vi "GDSLvClass_GetClassProviderInformation.vi"(0 "Class Refnum In":refnum<vi>, 5 "error in (no error)":errorcluster) -> (14 "Class Refnum Out":refnum<vi>, 15 "ClassProvider":T1, 19 "error out":errorcluster)   [LabVIEW 2020]
uses:
  GDSLvClass_ProviderTypes.ctl
  GDSLvClass_ClassTypeSettingNames.ctl
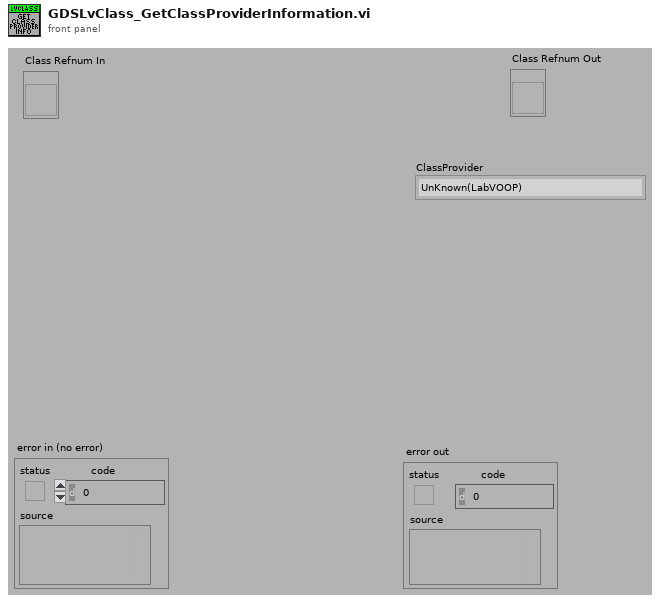
[diagram p1: front panel]
types:
  T1 = typedef "GDSLvClass_ProviderTypes.ctl" = enum16{"UnKnown(LabVOOP)", "Native", "EndevoGOOP3", "OpenG(RootObject)", "OpenG(OpenG_Object)", "EndevoGOOP4", "JKI1"}
  T2 = typedef "GDSLvClass_ClassTypeSettingNames.ctl" = enum16{"EndevoGOOP_ClassProvider", "EndevoGOOP_TemplateUsed", "EndevoGOOP_TemplateVersion", "EndevoGOOP_PlugIns", "EndevoGOOP_ConnectorPanePattern"}
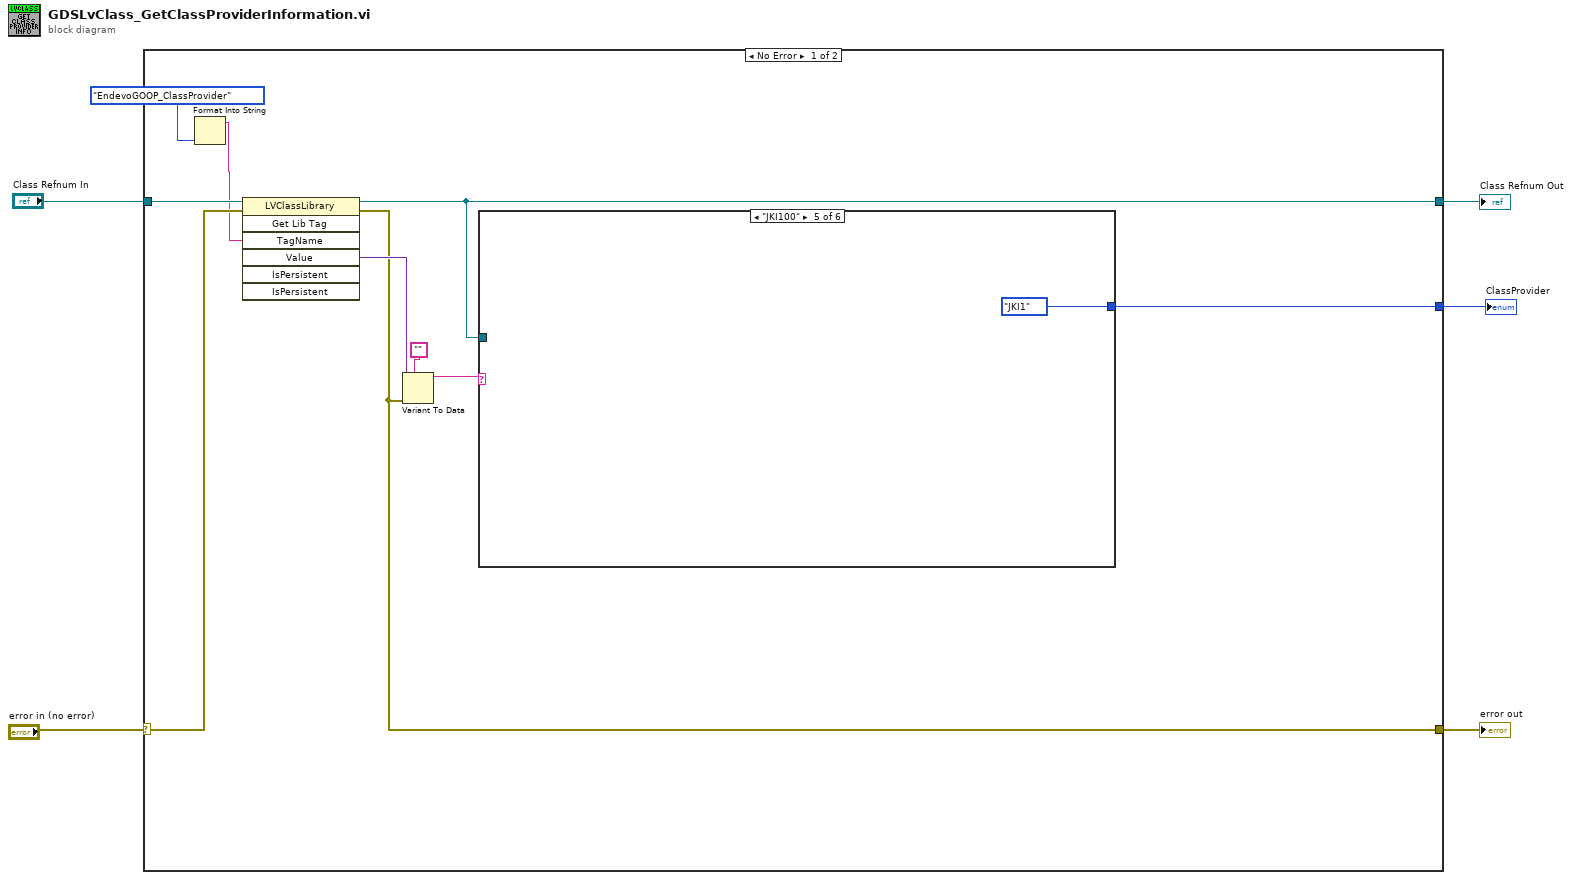
[diagram p0: block diagram]
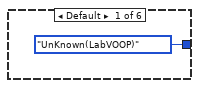
[diagram p2: hidden frame]
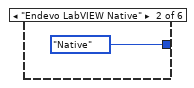
[diagram p3: hidden frame]
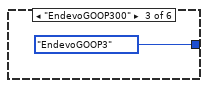
[diagram p4: hidden frame]
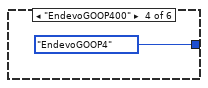
[diagram p5: hidden frame]
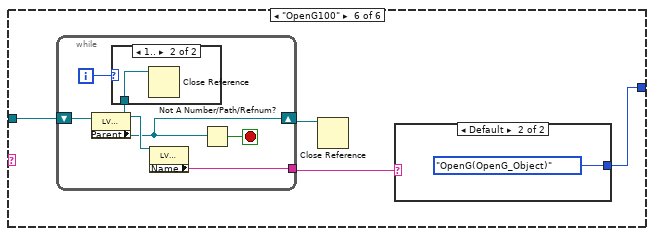
[diagram p6: hidden frame]
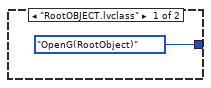
[diagram p7: hidden frame]
diagram:
  n1 = case shown="No Error" "error in (no error)" {
    selector: "error in (no error)" -> [w15 w35]
    tunnel: [w6 w35] -> w4
    tunnel: "Class Refnum In" -> [w13 w34]
    tunnel: [w7 w34] -> w2
    tunnel: [w8 _] -> w1
    frame No Error {
      n2 = Format Into String(GDSLvClass_ClassTypeSettingNames."EndevoGOOP_ClassProvider" ("ClassTypeSettingNames")) -> (resulting string=w11:string)  [unwired: 3 in, 1 out]
      n3 = invoke class="LVClassLibrary" method="Get Lib Tag"(reference=w13, error in=w15, "TagName"=w11) -> (reference out=w7:refnum<vi>, error out=w6:errorcluster, "Value"=w14:variant)  [unwired: 4 in, 4 out]
      n4 = Variant To Data(error in=w6, type="", Variant=w14) -> (data=w9:string)  [unwired: 1 out]
      n5 = case shown="\"JKI100\"" w9 {
        tunnel: [GDSLvClass_ProviderTypes."UnKnown(LabVOOP)" ("ClassProvider") GDSLvClass_ProviderTypes."Native" ("ClassProvider") GDSLvClass_ProviderTypes."EndevoGOOP3" ("ClassProvider") GDSLvClass_ProviderTypes."EndevoGOOP4" ("ClassProvider") GDSLvClass_ProviderTypes."JKI1" ("ClassProvider") w21] -> w8
        tunnel: w7 -> [_ _ _ _ _ w24]
        frame Default {
        }
        frame "Endevo LabVIEW Native" {
        }
        frame "EndevoGOOP300" {
        }
        frame "EndevoGOOP400" {
        }
        frame "JKI100" {
        }
        frame "OpenG100" {
          n6 = while {
            shift-right: [w28] -> w23
            shift-left: w24 -> [w32]
            tunnel: [w29] -> w22
            i -> [w31]
            stop <- w27 stop-if-true
            n7 = property class="LVClassLibrary"(reference=w32) -> (reference out=w30:refnum<vi>, "Parent"=w28:refnum<vi>)  [unwired: 1 in, 1 out]
            n8 = case shown="1.." w31 {
              tunnel: w30 -> [_ w33]
              frame Default {
              }
              frame 1.. {
                n9 = Close Reference(reference=w33) -> ()  [unwired: 1 in, 1 out]
              }
            }
            n10 = property class="LVClassLibrary"(reference=w30) -> ("Name"=w29:string)  [unwired: 1 in, 2 out]
            n11 = Not A Number/Path/Refnum?(number/path/refnum=w28) -> (NaN/Path/Refnum?=w27:bool)
          }
          n12 = Close Reference(reference=w23) -> ()  [unwired: 1 in, 1 out]
          n13 = case shown="Default" w22 {
            tunnel: [GDSLvClass_ProviderTypes."OpenG(RootObject)" ("ClassProvider") GDSLvClass_ProviderTypes."OpenG(OpenG_Object)" ("ClassProvider")] -> w21
            frame "RootOBJECT.lvclass" {
            }
            frame Default {
            }
          }
        }
      }
    }
    frame Error {
    }
  }
  "Class Refnum Out" <- w2
  "error out" <- w4
  "ClassProvider" <- w1
